vi "ZNB data loop.vi"(0 "VISA resource name":refnum<visa-resource-name>, 1 "Number of frequency points":i32, 2 "Frequencies":dbl[](array[numeric]), 3 "Delay Time":dbl, 4 "Output Port":i32, 5 "Input Port":i32, 6 "error in (no error)":errorcluster) -> (7 "error out":errorcluster, 20 "ReS":dbl[](array[numeric]), 21 "ImS":dbl[](array[numeric]), 22 "LinMagS":dbl[](array[numeric]), 23 "dBS":dbl[](array[numeric]), 24 "Phase":dbl[](array[numeric]), 25 "ReZ":dbl[](array[numeric]), 26 "ImZ":dbl[](array[numeric]), 27 "LinMagZ":dbl[](array[numeric]))   [LabVIEW 2015]
uses:
  <vilib>/express/express arith-compare/Formula/XNode/ExpressFormulaBlockNode.xnode
panel:
  out "VISA resource name out":refnum<visa-resource-name>
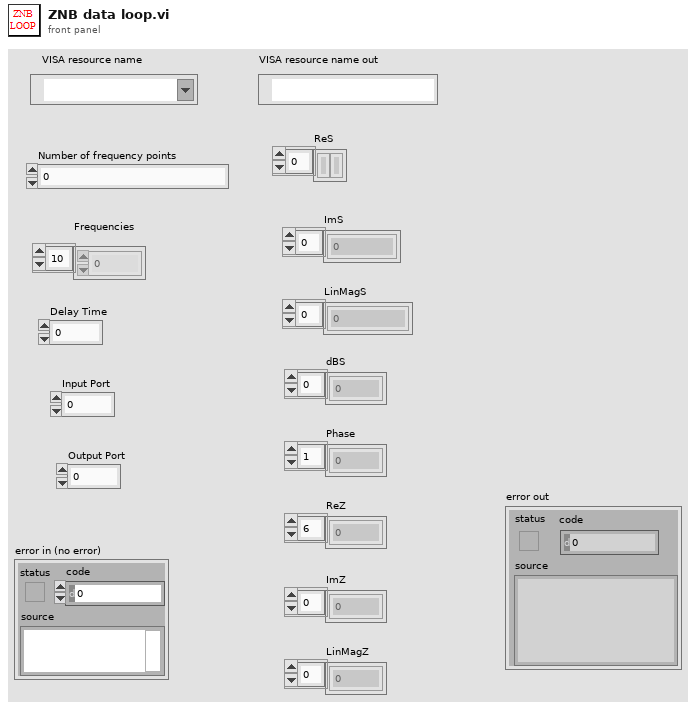
[diagram p1: front panel]
types:
  T1 = typedef "NI_Matrix.lvlib/RealMatrix.ctl" = dbl[][]
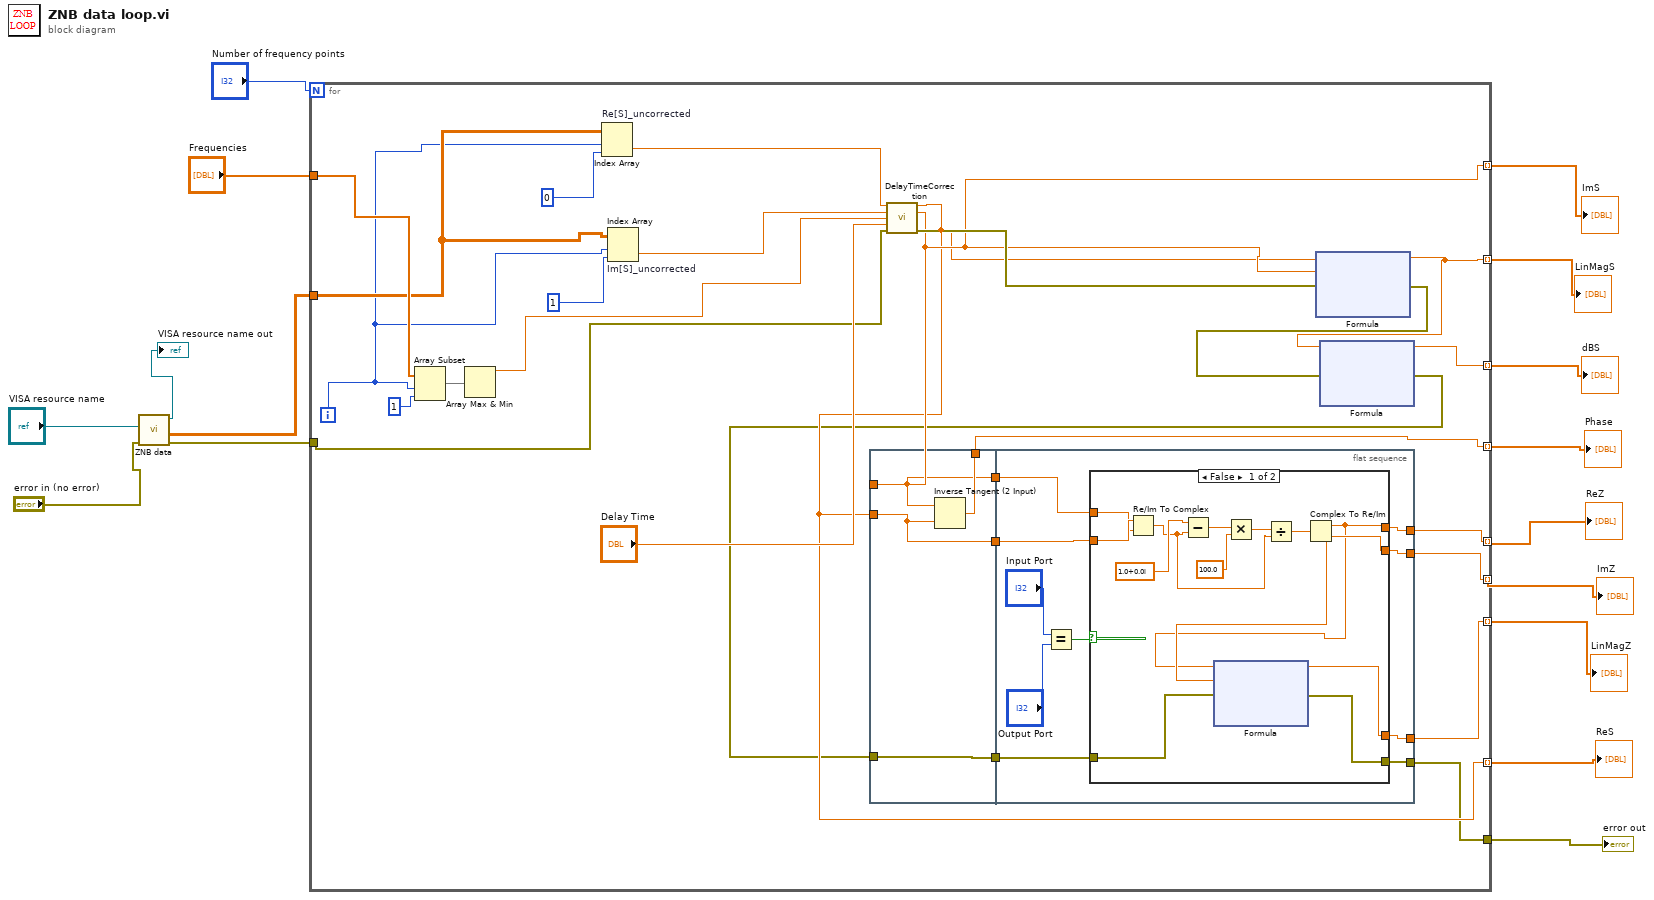
[diagram p0: block diagram]
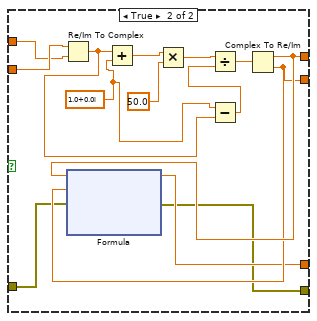
[diagram p2: hidden frame]
diagram:
  n1 = call "ZNB data.vi"("error in (no error)"="error in (no error)", "VISA resource name"="VISA resource name") -> ("error out"=w2:errorcluster, "Real Matrix"=w1:T1, "VISA resource name out"=→"VISA resource name out":refnum<visa-resource-name>)  [unwired: 7 in]
  n2 = for {
    N: "Number of frequency points" -> [_]
    tunnel: [w34] -> w15 mode=indexing
    tunnel: [w39] -> w14 mode=indexing
    tunnel: [w40] -> w13 mode=indexing
    tunnel: [w32] -> w12 mode=indexing
    tunnel: [w29] -> w11 mode=indexing
    tunnel: [w28] -> w10 mode=indexing
    tunnel: [w27] -> w9 mode=indexing
    tunnel: [w24] -> w8
    tunnel: "Frequencies" -> [w41]
    tunnel: [w33] -> w6 mode=indexing
    tunnel: w2 -> [w23]
    tunnel: w1 -> [w20]
    i -> [w17]
    n3 = Array Subset(array=w41, index=w17, length=1) -> (w42:dbl[])
    n4 = Array Max & Min(array=w42) -> (max value=w36:dbl)  [unwired: 3 out]
    n5 = Index Array "Re[S]_uncorrected"(array=w20, index (row)=w17, index (col)=0) -> (element=w19:dbl)
    n6 = Index Array "Im[S]_uncorrected"(array=w20, index (row)=w17, index (col)=1) -> (element=w18:dbl)
    n7 = flat-sequence {
      tunnel: w34 -> [w45]
      tunnel: w33 -> [w46]
      tunnel: [w47] -> w32
      tunnel: [w46] -> w31
      tunnel: [w45] -> w30
      tunnel: [w44] -> w26
      tunnel: w25 -> [w44]
      tunnel: w31 -> [w56]
      tunnel: w30 -> [w55]
      tunnel: [w54] -> w29
      tunnel: [w53] -> w28
      tunnel: [w52] -> w27
      tunnel: w26 -> [w51]
      tunnel: [w50] -> w24
      frame #0 {
        n8 = Inverse Tangent (2 Input)(1:w46, 2:w45) -> (0:w47:dbl)
      }
      frame #1 {
        n9 = Equal?(x="Input Port", y="Output Port") -> (x = y?=w57:bool)
        n10 = case shown="False" w57 {
          tunnel: w56 -> [w70 w88]
          tunnel: w55 -> [w69 w87]
          tunnel: [w61 w85] -> w54
          tunnel: [w62 w84] -> w53
          tunnel: [w60 w83] -> w52
          tunnel: w51 -> [w59 w82]
          tunnel: [w58 w81] -> w50
          frame False {
            n11 = Re/Im To Complex(1:w69, 2:w70) -> (0:w64:cdb)
            n12 = Subtract(x=cdb 1.0+0.0i, y=w64) -> (x-y=w67:cdb)
            n13 = Multiply(x=w67, y=100.0) -> (x*y=w65:cdb)
            n14 = Divide(x=w65, y=w64) -> (x/y=w63:cdb)
            n15 = Complex To Re/Im(x + iy=w63) -> (x=w61:dbl, y=w62:dbl)
            n16 = xnode "Formula"("ReS"=w61, "ImS"=w62, "error in (no error)"=w59) -> ("Result"=w60:dbl, "error out"=w58:errorcluster)
          }
          frame True {
            w91 = cdb 1.0+0.0i
            n17 = Re/Im To Complex(1:w87, 2:w88) -> (0:w90:cdb)
            n18 = Add(x=w90, y=w91) -> (x+y=w94:cdb)
            n19 = Multiply(x=w94, y=50.0) -> (x*y=w92:cdb)
            n20 = Subtract(x=w91, y=w90) -> (x-y=w89:cdb)
            n21 = Divide(x=w92, y=w89) -> (x/y=w86:cdb)
            n22 = Complex To Re/Im(x + iy=w86) -> (x=w85:dbl, y=w84:dbl)
            n23 = xnode "Formula"("ReS"=w85, "ImS"=w84, "error in (no error)"=w82) -> ("Result"=w83:dbl, "error out"=w81:errorcluster)
          }
        }
      }
    }
    n24 = call "DelayTimeCorrection.vi"("ReS"=w19, "ImS"=w18, "Frequency"=w36, "Dealy Time"="Delay Time", "error in (no error)"=w23) -> ("ReS_corrected"=w33:dbl, "ImS_corrected"=w34:dbl, "error out"=w37:errorcluster)  [unwired: 8 in]
    n25 = xnode "Formula"("ReS"=w33, "ImS"=w34, "error in (no error)"=w37) -> ("Result"=w39:dbl, "error out"=w38:errorcluster)
    n26 = xnode "Formula"("LinMag"=w39, "error in (no error)"=w38) -> ("Result"=w40:dbl, "error out"=w25:errorcluster)
  }
  "error out" <- w8
  "ReS" <- w6
  "ImS" <- w15
  "LinMagS" <- w14
  "dBS" <- w13
  "Phase" <- w12
  "ReZ" <- w11
  "ImZ" <- w10
  "LinMagZ" <- w9
